vi "__Recursive File List with Exclude Option.vi"(4 "Folders to Exclude\nREP ( ^[_.] as Default)\nempty to disable this feature":string="^[_.]", 6 "pattern":string, 8 "error in (no error)":errorcluster, 11 "Folder Path":path) -> (0 "error out":errorcluster, 1 "Number of Files":i32, 2 "All Files in Dir":path[](array[path]), 3 "dup Folder Path":path, 5 "All Folders":path[](array[path]))   [LabVIEW 2019, in "LabVIEW-ProviderShell.lvlib"]
doc: "Lists the contents of a folder or LLB.NEVSTOP-Programming-Palette 2022.3.9.1\nNEVSTOP - NEVSTOP\nCopyright (c) 2022, NEVSTOP"
uses:
  LabVIEW-ProviderShell.lvlib
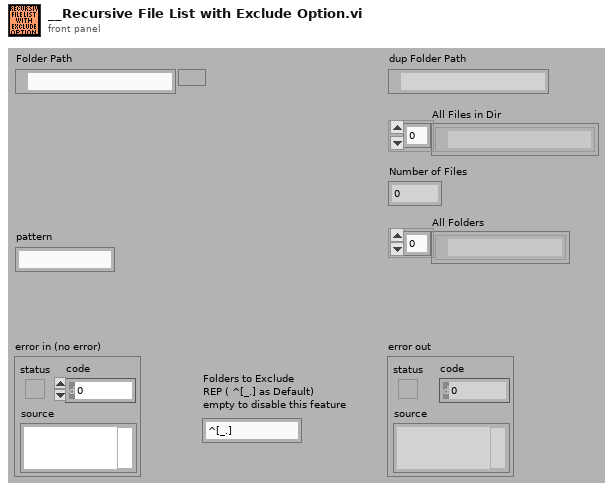
[diagram p1: front panel]
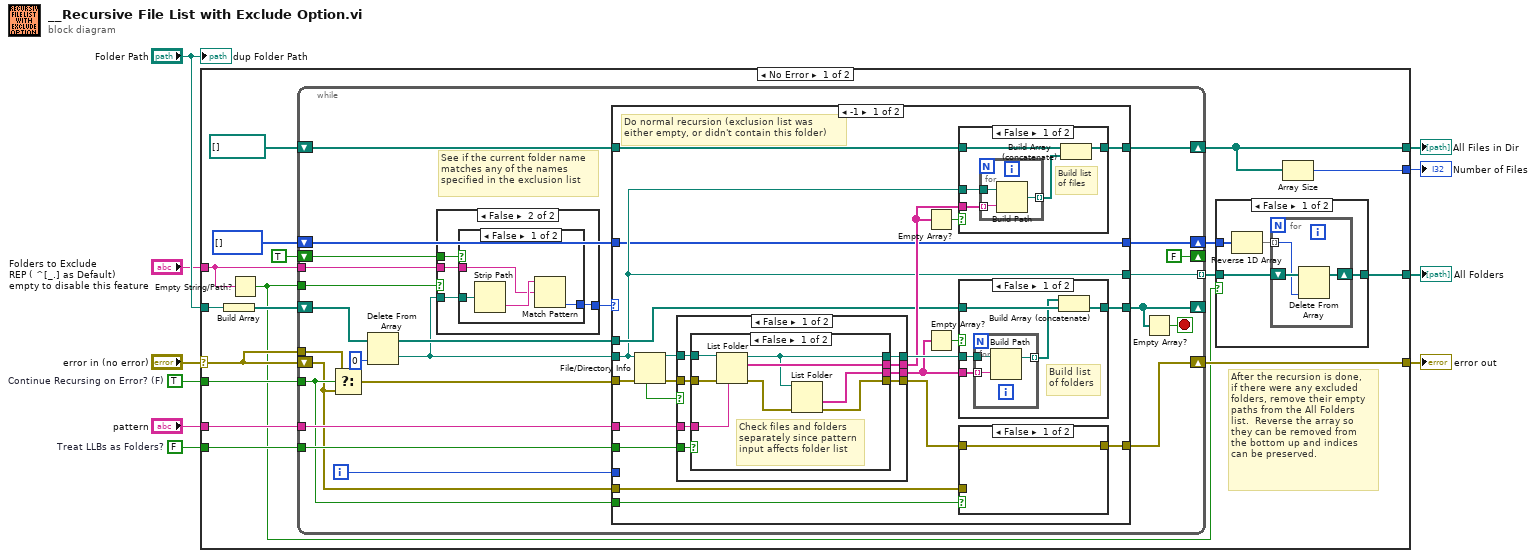
[diagram p0: block diagram]
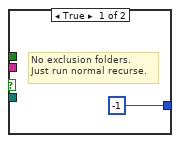
[diagram p3: hidden frame]
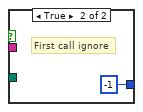
[diagram p4: hidden frame]
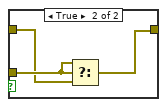
[diagram p6: hidden frame]
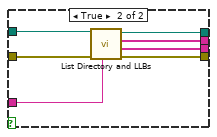
[diagram p7: hidden frame]
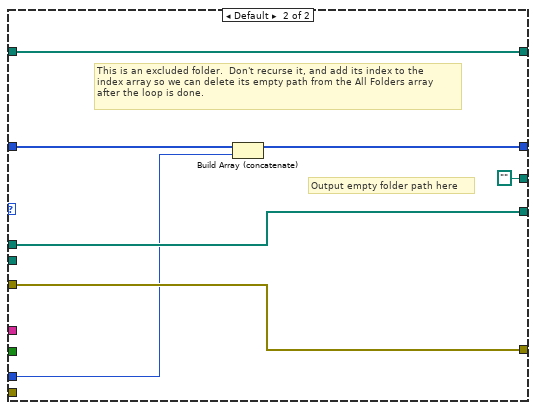
[diagram p10: hidden frame]
diagram:
  w2 = TRUE  # Continue Recursing on Error? (F)
  w6 = FALSE  # Treat LLBs as Folders?
  n1 = case shown="No Error" "error in (no error)" {
    selector: "error in (no error)" -> [w18 w145]
    tunnel: "Folder Path" -> [w27 _]
    tunnel: [w21 _] -> w10
    tunnel: [w20 _] -> w9
    tunnel: [w22 w145] -> w8
    tunnel: w6 -> [w24 _]
    tunnel: [w13 _] -> w5
    tunnel: "pattern" -> [w23 _]
    tunnel: w2 -> [w19 _]
    tunnel: "Folders to Exclude\nREP ( ^[_.] as Default)\nempty to disable this feature" -> [w16 _]
    frame No Error {
      # "After the recursion is done,\nif there were any excluded\nfolders, remove their empty\npaths from the All Folders\nlist.  Reverse the array so\nthey can be removed from\nthe bottom up and indices\ncan be preserved."
      n2 = Build Array(w27) -> (w26:path[])
      n3 = Empty String/Path?(string/path=w16) -> (empty?=w14:bool)
      n4 = while {
        shift-left: path[] [] ("Array Constant") -> [w57]
        shift-right: [w59] -> w21
        shift-left: w26 -> [w58]
        shift-right: [w54] -> _
        shift-right: [w48] -> w22
        shift-left: w18 -> [w47]
        tunnel: w24 -> [w56]
        tunnel: [w44] -> w15 mode=indexing
        tunnel: w23 -> [w55]
        tunnel: w19 -> [w49]
        tunnel: w18 -> [w50]
        tunnel: w16 -> [w40]
        shift-right: [w43] -> w12
        shift-left: i32[] [] -> [w45]
        tunnel: w14 -> [w41]
        shift-right: [FALSE] -> _
        shift-left: TRUE -> [w36]
        i -> [w42]
        stop <- w53 stop-if-true
        # "See if the current folder name\nmatches any of the names\nspecified in the exclusion list"
        n5 = Select(t=w50, s=w49, f=w47) -> (s? t:f=w51:errorcluster)
        n6 = Delete From Array(array=w58, index=0) -> (deleted portion=w39:path, array with subset deleted=w46:path[])  [unwired: 1 in]
        n7 = case shown="False" w41 {
          tunnel: w40 -> [_ w62]
          tunnel: w39 -> [_ w64]
          tunnel: [-1 ("index of element") w63] -> w38
          tunnel: w36 -> [_ w61]
          frame True {
            # "No exclusion folders.\nJust run normal recurse."
          }
          frame False {
            n8 = case shown="False" w61 {
              tunnel: w64 -> [w68 _]
              tunnel: [w67 -1 ("offset past match")] -> w63
              tunnel: w62 -> [w65 _]
              frame False {
                n9 = Strip Path(path=w68) -> (name=w66:string)  [unwired: 1 out]
                n10 = Match Pattern(string=w66, regular expression=w65) -> (offset past match=w67:i32)  [unwired: 1 in, 3 out]
              }
              frame True {
                # "First call ignore"
              }
            }
          }
        }
        n11 = case shown="-1" w38 {
          tunnel: [w90 w144] -> w59
          tunnel: w57 -> [w89 w144]
          tunnel: w56 -> [w87 _]
          tunnel: w55 -> [w86 _]
          tunnel: [w83 w143] -> w54
          tunnel: w39 -> [w71 _]
          tunnel: w51 -> [w79 w142]
          tunnel: w49 -> [w77 _]
          tunnel: [w76 w142] -> w48
          tunnel: w47 -> [w75 _]
          tunnel: w46 -> [w72 w143]
          tunnel: w45 -> [w70 w141]
          tunnel: [w71 path ""] -> w44
          tunnel: [w70 w140] -> w43
          tunnel: w42 -> [_ w139]
          frame -1 {
            # "Do normal recursion (exclusion list was\neither empty, or didn't contain this folder)"
            n12 = File/Directory Info(path=w71, error in=w79) -> (path out=w81:path, error out=w82:errorcluster, shortcut=w80:bool)  [unwired: 4 out]
            n13 = case shown="False" w80 {
              tunnel: [w111 _] -> w73
              tunnel: [w110 w128] -> w88
              tunnel: [w109 w127] -> w78
              tunnel: w87 -> [w108 _]
              tunnel: w86 -> [w107 _]
              tunnel: [w106 _] -> w85
              tunnel: w82 -> [w105 w127]
              tunnel: w81 -> [w104 w128]
              frame False {
                n14 = case shown="False" w108 {
                  tunnel: [w119 w123] -> w111
                  tunnel: [w113 w122] -> w106
                  tunnel: w104 -> [w118 w126]
                  tunnel: [w112 w124] -> w110
                  tunnel: [w114 w121] -> w109
                  tunnel: w105 -> [w117 w125]
                  tunnel: w107 -> [w116 w120]
                  frame False {
                    # "Check files and folders\nseparately since pattern\ninput affects folder list"
                    n15 = List Folder(path=w118, pattern=w116, error in=w117) -> (path out=w112:path, filenames=w119:string[], error out=w115:errorcluster)  [unwired: 2 out]
                    n16 = List Folder(path=w112, error in=w115) -> (folder names=w113:string[], error out=w114:errorcluster)  [unwired: 4 out]
                  }
                  frame True {
                    n17 = call <vilib>:"List Directory and LLBs.vi"("pattern"=w120, "error in (no error)"=w125, "Folder Path"=w126) -> ("error out"=w121:errorcluster, "Folders and LLBs"=w122:string[], "Files sans LLBs"=w123:string[], "dup Folder Path"=w124:path)  [unwired: 5 out]
                  }
                }
              }
              frame True {
                # "Do not attempt to recurse the contents\nof folder shortcuts"
              }
            }
            n18 = Empty Array?(array=w73) -> (empty?=w74:bool)
            n19 = Empty Array?(array=w85) -> (empty?=w84:bool)
            n20 = case shown="False" w74 {
              tunnel: [w95 w99] -> w90
              tunnel: w73 -> [w94 _]
              tunnel: w89 -> [w93 w99]
              tunnel: w71 -> [w91 _]
              frame False {
                # "Build list of files"
                n21 = for {
                  tunnel: w94 -> [w97] mode=indexing
                  tunnel: w91 -> [w98]
                  tunnel: [w96] -> w92 mode=indexing
                  n22 = Build Path(base path=w98, name or relative path=w97) -> (appended path=w96:path)
                }
                n23 = Build Array (concatenate)(w93, w92) -> (w95:path[])
              }
              frame True {
              }
            }
            n24 = case shown="False" w84 {
              tunnel: w72 -> [w131 w137]
              tunnel: [w132 w137] -> w83
              tunnel: w88 -> [w133 _]
              tunnel: w85 -> [w129 _]
              frame False {
                # "Build list\nof folders"
                n25 = for {
                  tunnel: w133 -> [w136]
                  tunnel: [w135] -> w130 mode=indexing
                  tunnel: w129 -> [w134] mode=indexing
                  n26 = Build Path(base path=w136, name or relative path=w134) -> (appended path=w135:path)
                }
                n27 = Build Array (concatenate)(w130, w131) -> (w132:path[])
              }
              frame True {
              }
            }
            n28 = case shown="False" w77 {
              tunnel: w78 -> [w100 w102]
              tunnel: [w100 w101] -> w76
              tunnel: w75 -> [_ w103]
              frame False {
              }
              frame True {
                n29 = Select(t=w103, s=w103, f=w102) -> (s? t:f=w101:errorcluster)
              }
            }
          }
          frame Default {
            # "Output empty folder path here"
            # "This is an excluded folder.  Don't recurse it, and add its index to the\nindex array so we can delete its empty path from the All Folders array\nafter the loop is done."
            n30 = Build Array (concatenate)(w141, w139) -> (w140:i32[])
          }
        }
        n31 = Empty Array?(array=w54) -> (empty?=w53:bool)
      }
      n32 = case shown="False" w14 {
        tunnel: w15 -> [w30 w35]
        tunnel: [w29 w35] -> w13
        tunnel: w12 -> [w31 _]
        frame False {
          n33 = Reverse 1D Array(array=w31) -> (reversed array=w28:i32[])
          n34 = for {
            shift-right: [w33] -> w29
            shift-left: w30 -> [w34]
            tunnel: w28 -> [w32] mode=indexing
            n35 = Delete From Array(array=w34, index=w32) -> (array with subset deleted=w33:path[])  [unwired: 1 in, 1 out]
          }
        }
        frame True {
          # "No excluded folders.\nDon't run the code that\ndeletes excluded folder\nindices."
        }
      }
      n36 = Array Size(array=w21) -> (size(s)=w20:i32)
    }
    frame Error {
    }
  }
  "All Files in Dir" <- w10
  "Number of Files" <- w9
  "error out" <- w8
  "All Folders" <- w5
  "dup Folder Path" <- "Folder Path"
